vi "DB_Close.vi"(8 "error in (no error)":errorcluster, 11 "SQLite Connection in":refnum<class "Connection.lvclass">) -> (0 "error out":errorcluster)   [LabVIEW 2020]
uses:
  <vilib>/drjdpowell/SQLite Library/SQL Connection/Connection.lvclass
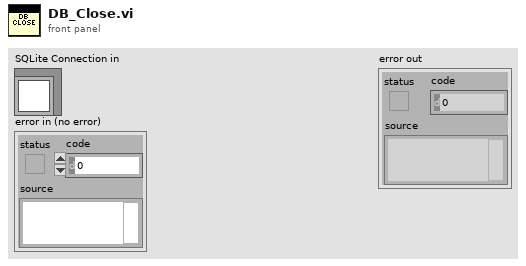
[diagram p1: front panel]
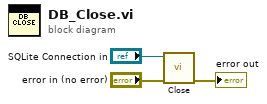
[diagram p0: block diagram]
diagram:
  n1 = call-dynamic "Close.vi"("error in (no error)"="error in (no error)", "SQLite Connection in"="SQLite Connection in") -> ("error out"=→"error out":errorcluster)  [unwired: 9 in]
